vi "Test_Code.vi"() -> ()   [LabVIEW 2015]
uses:
  <instrlib>/Agilent N6700 Series/Agilent N6700 Series.lvlib
  <vilib>/Utility/NIReport.llb/NI_report.lvclass
  Global 5.vi
  <vilib>/Instr/_visa.llb/Select Event Type.ctl
  <vilib>/Instr/_visa.llb/VISA Configure Serial Port (Instr).vi
  Serial - XON-XOFF Characters.ctl
  Serial - ASCII Characters.ctl
  Serial - Settings.ctl
panel:
  in  "report file path":path=path "C:/Users/Tulio/Documents/Testes/Backup excel/backup excel.xlsx"
  out "Hour":i32
  out "Minute":i32
  out "Second":i32
  out "Fractional Second":dbl format="%#.4g"
  in  "Negative Voltage Limit (0.0 volts)":dbl format="%^.3e"
  out "Waveform Graph":dbl[](graph)
  out "Count":i32
  out "read buffer":string
  in  "Read Count":u32=1000
  out "Action":string
  in  "Termination Character":u8=10 format="%.0x"
  in  "End Write on Termination Character?":bool=TRUE
  in  "VISA resource name 2":refnum<visa-resource-name>="COM27"
  in  "XON/XOFF Characters":T1={"XON"=enum."DC1", "XOFF"=enum."DC3"}
  in  "Serial Settings":T3={"baud rate"=9600, "data bits"=8, "parity"=enum."None", "stop bits"=10, "flow control"=0} {"flow control" items=["None"=0, "XON/XOFF"=1, "RTS/CTS"=2, "DTR/DSR"=4]; "stop bits" items=["1.0"=10, "1.5"=15, "2.0"=20]; "data bits" min=5 max=8 step=1; "baud rate" items=["75"=75, "110"=110, "134"=134, "150"=150, "300"=300, "600"=600, "1200"=1200, "1800"=1800, "2400"=2400, "4800"=4800, "7200"=7200, "9600"=9600, "14400"=14400, "19200"=19200, "28800"=28800, "38400"=38400, "56000"=56000, "57600"=57600, "115200"=115200, "128000"=128000, "230400"=230400]}
  in  "End Read on Termination Character?":bool=TRUE
  in  "Start":bool
  in  "Priority (1: Voltage)":i32(ring) items=["Voltage"=1, "Current"=0]
  out "Current Measurement":dbl format="%^.3e"
  in  "Positive Voltage Limit  (5.0 V)":dbl=5.0 format="%^.3e"
  in  "Channel Name (1)":string="4"
  in  "VISA resource name":refnum<visa-resource-name>="USB0::0x0957::0x0F07::MY53002228::INSTR"
  in  "stop":bool
  # "SERIAL"
  # "POWER ANALYZER"
  # "EXCEL"
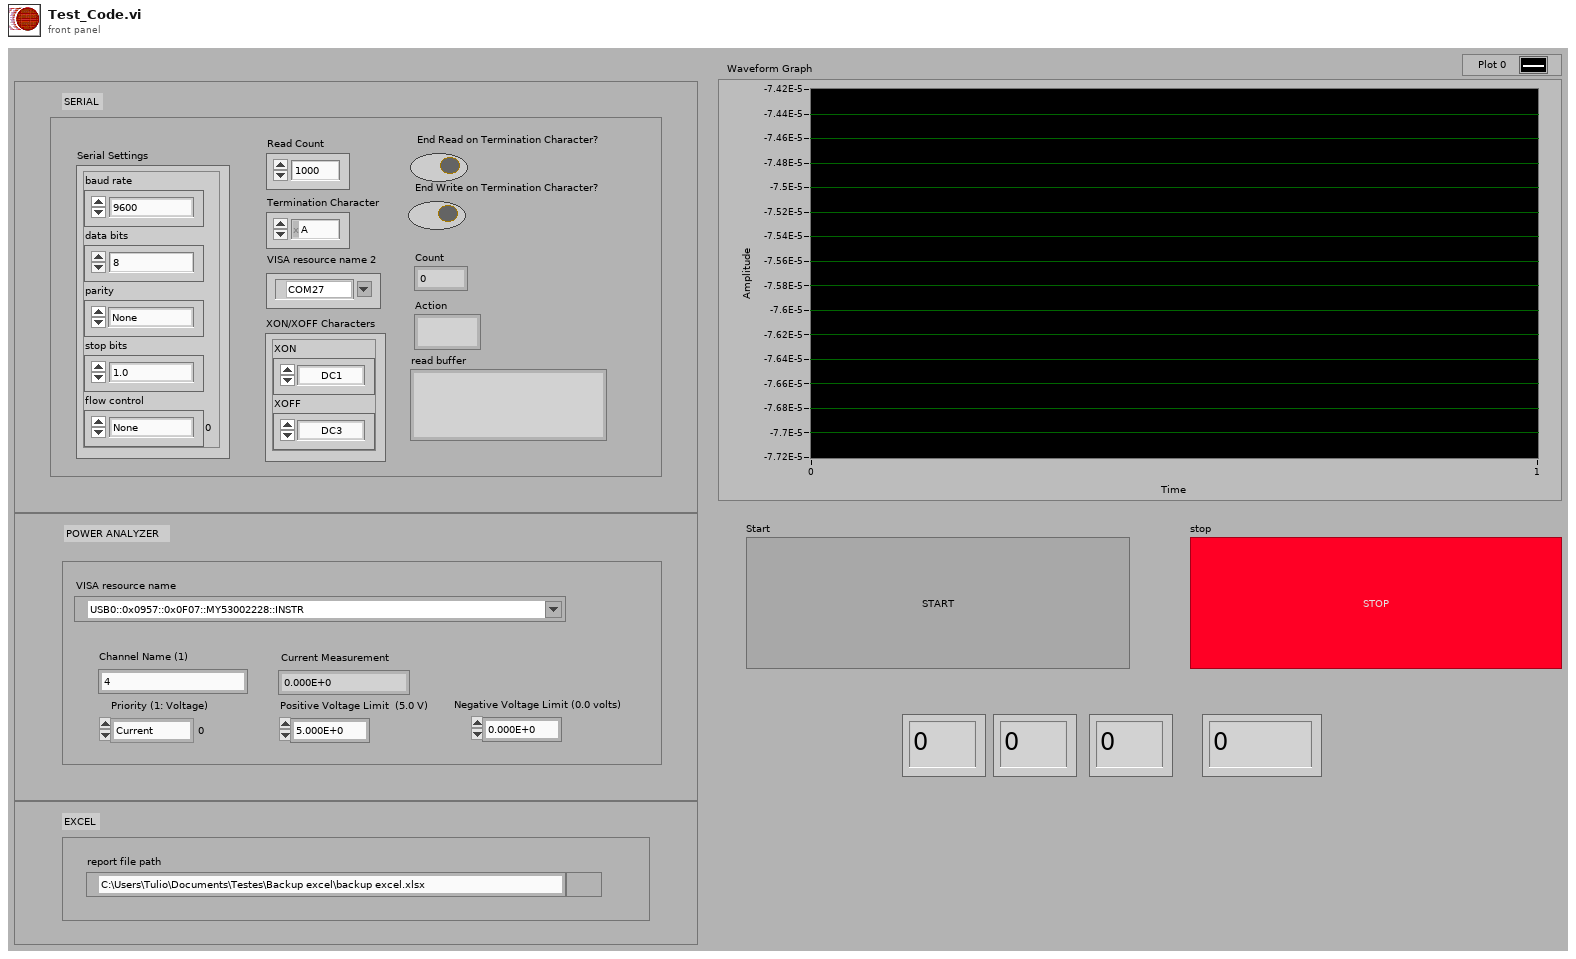
[diagram p1: front panel]
types:
  T1 = typedef "Serial - XON-XOFF Characters.ctl" = cluster{"XON":T2, "XOFF":T2}
  T2 = typedef "Serial - ASCII Characters.ctl" = enum16{"NUL", "SOH", "STX", "ETX", "EOT", "ENQ", "ACK", "BEL", "BS", "HT", "LF", "VT", "FF", "CR", "SO", "SI", "DLE", "DC1", "DC2", "DC3", "DC4", "NAK", "SYN", "ETB", "CAN", "EM", "SUB", "ESC", "FS", "GS", "RS", "US", "SP", "!", "\"", "#", "$", "%", "&", "'", "(", ")", "*", "+", ",", "- (-)", ".", "/", "0", "1", "2", "3", "4", "5", "6", "7", "8", "9", ":", ";", "<", "=", ">", "?", "@", "A", "B", "C", "D", "E", "F", "G", "H", "I", "J", "K", "L", "M", "N", "O", "P", "Q", "R", "S", "T", "U", "V", "W", "X", "Y", "Z", "[", "\\", "]", "^", "_", "`", "a", "b", "c", "d", "e", "f", "g", "h", "i", "j", "k", "l", "m", "n", "o", "p", "q", "r", "s", "t", "u", "v", "w", "x", "y", "z", "{", "|", "}", "~"}
  T3 = typedef "Serial - Settings.ctl" = cluster{"baud rate":u32, "data bits":u16, "parity":enum16{"None", "Odd", "Even", "Mark", "Space"}, "stop bits":u16, "flow control":u16}
  T4 = enum16{"Standard Report", "HTML", "Word", "Excel"}
  T5 = typedef "Select Event Type.ctl" = u32
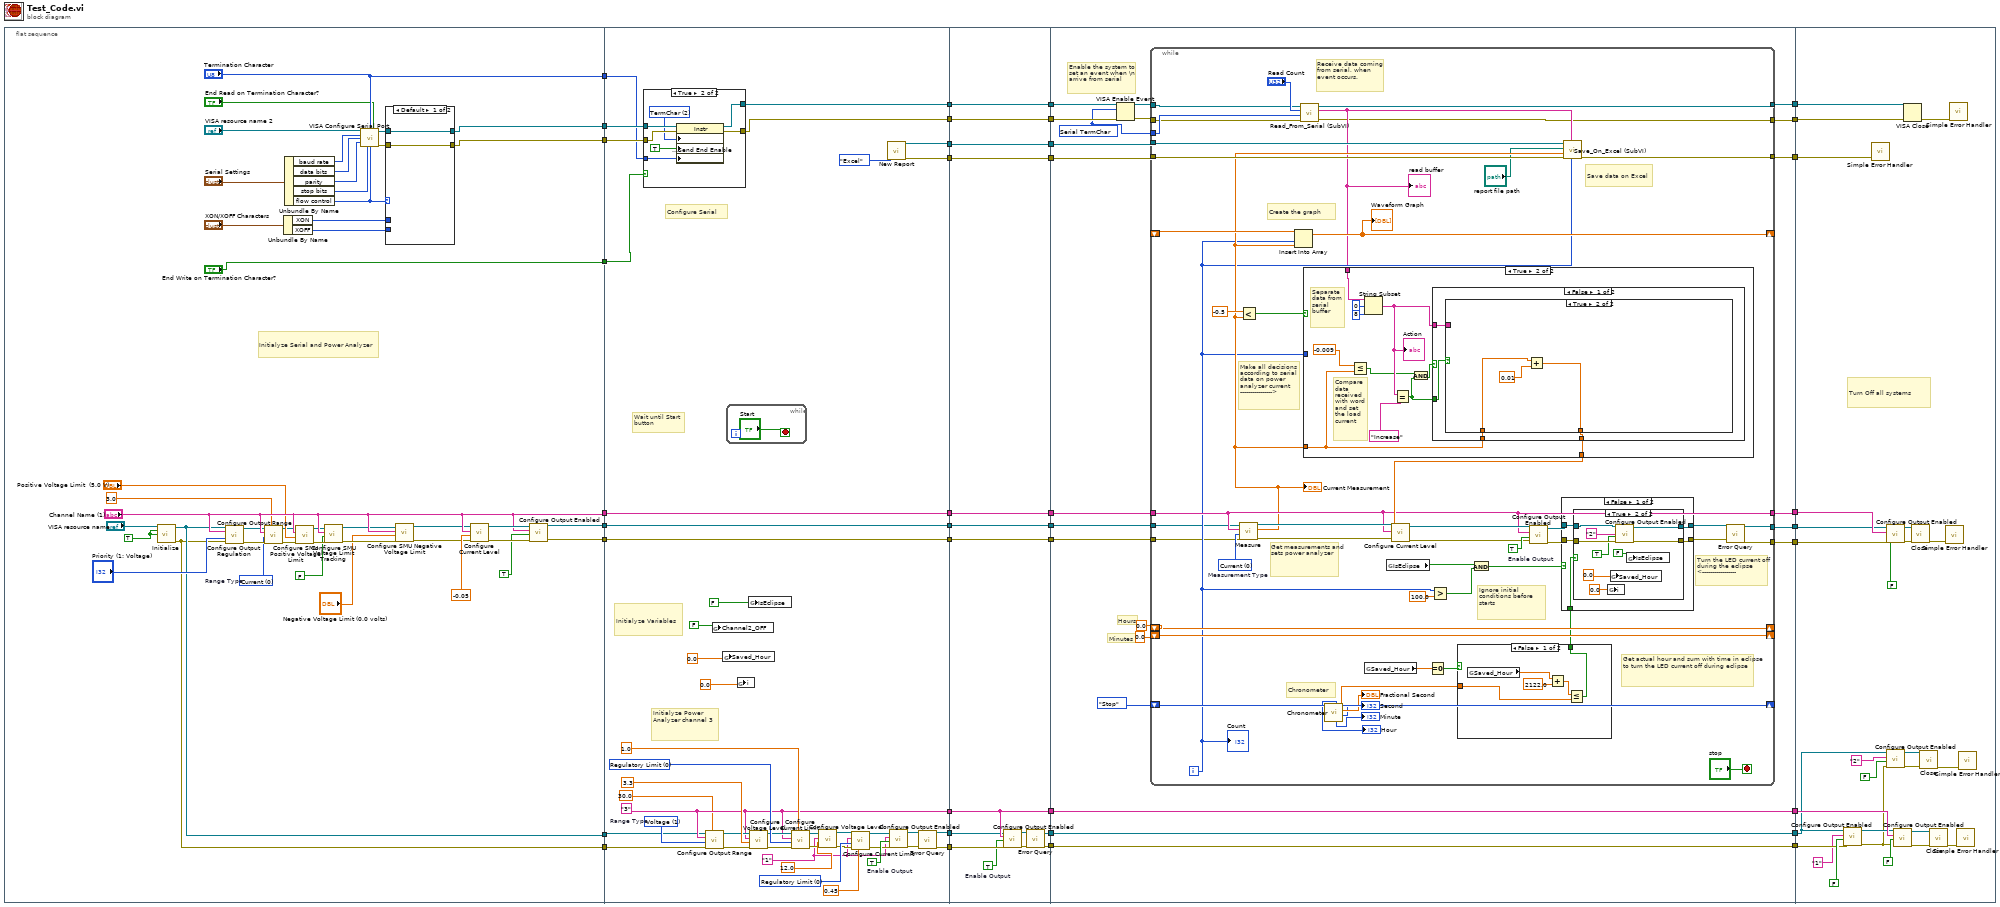
[diagram p0: block diagram]
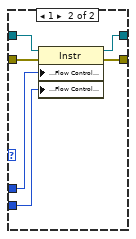
[diagram p2: hidden frame]
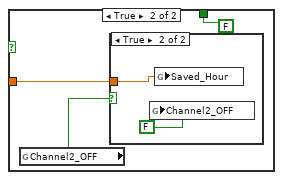
[diagram p4: hidden frame]
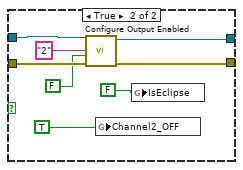
[diagram p7: hidden frame]
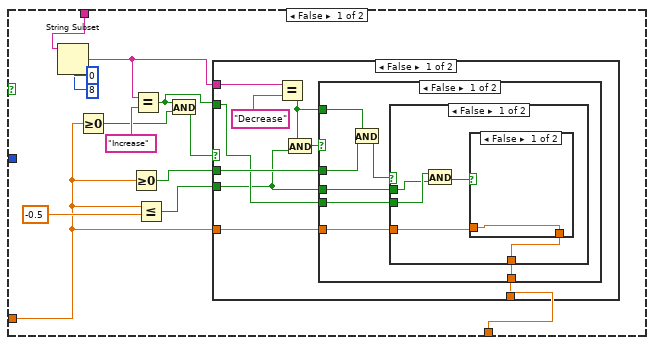
[diagram p8: hidden frame]
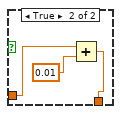
[diagram p9: hidden frame]
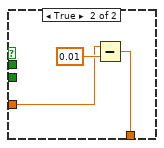
[diagram p10: hidden frame]
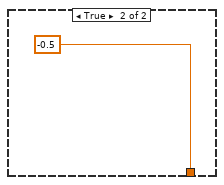
[diagram p11: hidden frame]
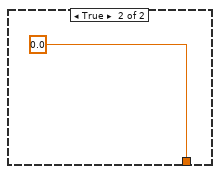
[diagram p12: hidden frame]
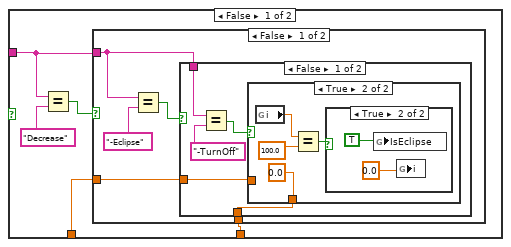
[diagram p13: hidden frame]
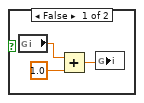
[diagram p15: hidden frame]
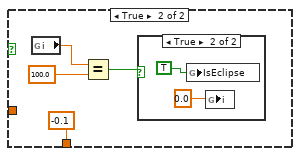
[diagram p16: hidden frame]
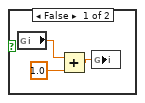
[diagram p17: hidden frame]
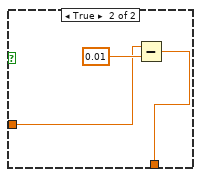
[diagram p18: hidden frame]
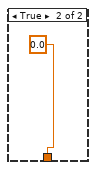
[diagram p19: hidden frame]
diagram:
  n1 = flat-sequence {
    tunnel: ["Channel Name (1)"] -> w38
    tunnel: [w80] -> w37
    tunnel: [w79] -> w36
    tunnel: [w40] -> w35
    tunnel: [w39] -> w34
    tunnel: [w76] -> w25
    tunnel: [w75] -> w24
    tunnel: ["End Write on Termination Character?"] -> w23
    tunnel: ["Termination Character"] -> w22
    tunnel: [w111] -> w20
    tunnel: [w133] -> w18
    tunnel: w38 -> [w133]
    tunnel: [w132] -> w16
    tunnel: w37 -> [w132]
    tunnel: [w131] -> w14
    tunnel: w36 -> [w131]
    tunnel: w35 -> [w112]
    tunnel: w34 -> [w114]
    tunnel: [w122] -> w11
    tunnel: w25 -> [w121]
    tunnel: w24 -> [w120]
    tunnel: w23 -> [w119]
    tunnel: w22 -> [w118]
    tunnel: [w110] -> w9
    tunnel: [w116] -> w7
    tunnel: [w115] -> w5
    tunnel: [w92] -> w2
    tunnel: [w91] -> w1
    tunnel: w20 -> [w158]
    tunnel: [w158] -> w19
    tunnel: w18 -> [w157]
    tunnel: [w157] -> w17
    tunnel: w16 -> [w156]
    tunnel: [w156] -> w15
    tunnel: w14 -> [w155]
    tunnel: [w155] -> w13
    tunnel: [w150] -> w12
    tunnel: w11 -> [w145]
    tunnel: [w145] -> w10
    tunnel: w9 -> [w154]
    tunnel: [w154] -> w8
    tunnel: w7 -> [w153]
    tunnel: [w153] -> w6
    tunnel: w5 -> [w152]
    tunnel: [w152] -> w4
    tunnel: [w151] -> w3
    tunnel: w2 -> [w144]
    tunnel: w1 -> [w147]
    tunnel: w19 -> [w164]
    tunnel: w17 -> [w180]
    tunnel: w15 -> [w179]
    tunnel: w13 -> [w178]
    tunnel: [w177] -> w33
    tunnel: [w176] -> w32
    tunnel: [w175] -> w31
    tunnel: [w174] -> w30
    tunnel: [w173] -> w29
    tunnel: w12 -> [w173]
    tunnel: w10 -> [w172]
    tunnel: [w172] -> w28
    tunnel: [w159] -> w27
    tunnel: [w171] -> w26
    tunnel: w8 -> [w163]
    tunnel: w6 -> [w167]
    tunnel: w4 -> [w166]
    tunnel: [w165] -> w21
    tunnel: w3 -> [w174]
    tunnel: w26 -> [w378]
    tunnel: w27 -> [w379]
    tunnel: w28 -> [w381]
    tunnel: w29 -> [w366]
    tunnel: w30 -> [w368]
    tunnel: w31 -> [w386]
    tunnel: w32 -> [w371]
    tunnel: w33 -> [w370]
    tunnel: w21 -> [w372]
    frame #0 {
      w65 = TRUE ("Reset? (T: Yes)")
      w64 = 0 items=["Voltage"=1, "Current"=0]  # Range Type
      # "Initialyze Serial and Power Analyzer"
      n2 = call <instrlib>:"Initialize.vi"("VISA resource name"="VISA resource name", "ID Query? (T: Yes)"=w65, "Reset? (T: Yes)"=w65) -> ("VISA resource name out"=w40:refnum<visa-resource-name>, "error out"=w39:errorcluster)  [unwired: 11 in]
      n3 = call <instrlib>:"Configure Output Regulation.vi"("VISA resource name"=w40, "Channel Name (1)"="Channel Name (1)", "Output Regulation Priority (1: Voltage)"="Priority (1: Voltage)", "error in (no error)"=w39) -> ("VISA resource name out"=w66:refnum<visa-resource-name>, "error out"=w67:errorcluster)  [unwired: 10 in]
      n4 = call <instrlib>:"Configure Output Range.vi"("Range (0.0)"=3.0, "error in (no error)"=w67, "Range Type (1: Voltage)"=w64, "Channel Name (1)"="Channel Name (1)", "VISA resource name"=w66) -> ("error out"=w69:errorcluster, "VISA resource name out"=w68:refnum<visa-resource-name>)  [unwired: 5 in]
      n5 = Unbundle By Name("XON/XOFF Characters") -> ("XON"=w57:T2, "XOFF"=w58:T2)
      n6 = Unbundle By Name("Serial Settings") -> ("baud rate"=w53:u32, "data bits"=w52:u16, "parity"=w51:enum16{"None", "Odd", "Even", "Mark", "Space"}, "stop bits"=w50:u16, "flow control"=w56:u16)
      n7 = call <instrlib>:"Configure SMU Positive Voltage Limit.vi"("error in (no error)"=w69, "Positive Voltage Limit (0.0 volts)"="Positive Voltage Limit  (5.0 V)", "Channel Name (1)"="Channel Name (1)", "VISA resource name"=w68) -> ("error out"=w71:errorcluster, "VISA resource name out"=w70:refnum<visa-resource-name>)  [unwired: 6 in]
      n8 = call <instrlib>:"Configure SMU Voltage Limit Tracking.vi"("error in (no error)"=w71, "Enable Voltage Limit Tracking (False)"=FALSE, "Channel Name (1)"="Channel Name (1)", "VISA resource name"=w70) -> ("error out"=w44:errorcluster, "VISA resource name out"=w45:refnum<visa-resource-name>)  [unwired: 6 in]
      n9 = call-poly "VISA Configure Serial Port"("VISA resource name"="VISA resource name 2", "termination char\n(0xA = '\\n' = LF)"="Termination Character", "Enable Termination\nChar (T)"="End Read on Termination Character?", "baud rate (9600)"=w53, "data bits (8)"=w52, "parity (0:none)"=w51, "stop bits (10: 1 bit)"=w50, "flow control (0:none)"=w56) -> ("VISA resource name out"=w49:refnum<visa-resource-name>, "error out"=w48:errorcluster)  [unwired: 2 in, 4 out]
      n10 = case shown="Default" w56 {
        tunnel: [w83 w90] -> w75
        tunnel: [w84 w89] -> w76
        tunnel: w48 -> [w83 w88]
        tunnel: w49 -> [w84 w87]
        tunnel: w57 -> [_ w86]
        tunnel: w58 -> [_ w85]
        frame Default {
        }
        frame 1 {
          n11 = property class="Instr"(reference=w87, error in=w88, "Serial Settings:Flow Control XON Character"=w86, "Serial Settings:Flow Control XOFF Character"=w85) -> (reference out=w89:refnum<visa-resource-name>, error out=w90:errorcluster)
        }
      }
      n12 = call <instrlib>:"Configure SMU Negative Voltage Limit.vi"("error in (no error)"=w44, "Negative Voltage Limit (0.0 volts)"="Negative Voltage Limit (0.0 volts)", "Channel Name (1)"="Channel Name (1)", "VISA resource name"=w45) -> ("error out"=w41:errorcluster, "VISA resource name out"=w42:refnum<visa-resource-name>)  [unwired: 6 in]
      n13 = call <instrlib>:"Configure Current Level.vi"("error in (no error)"=w41, "Level  (0.0 A)"=-0.05, "Channel Name (1)"="Channel Name (1)", "VISA resource name"=w42) -> ("error out"=w81:errorcluster, "VISA resource name out"=w82:refnum<visa-resource-name>)  [unwired: 6 in]
      n14 = call <instrlib>:"Configure Output Enabled.vi"("error in (no error)"=w81, "Enable Output (False)"=TRUE, "Channel Name (1)"="Channel Name (1)", "VISA resource name"=w82) -> ("error out"=w79:errorcluster, "VISA resource name out"=w80:refnum<visa-resource-name>)  [unwired: 6 in]
    }
    frame #1 {
      w94 = "1" ("Channel Name (1)")
      w102 = 0 items=["Regulatory Limit", "Trip Limit"] ("Behavior (0: Regulatory Limit)")
      w104 = TRUE  # Enable Output
      w122 = "3" ("Channel Name (1)")
      w129 = 0 items=["Regulatory Limit", "Trip Limit"] ("Behavior (0: Regulatory Limit)")
      w125 = 1 items=["Voltage"=1, "Current"=0]  # Range Type
      # "Initialyze Power Analyzer channel 3"
      # "Initialyze Variables"
      # "Wait until Start button"
      # "Configure Serial"
      n15 = case shown="True" w119 {
        tunnel: w121 -> [w134 w142]
        tunnel: w120 -> [w135 w141]
        tunnel: [w134 w140] -> w111
        tunnel: [w135 w139] -> w110
        tunnel: w118 -> [_ w137]
        frame False {
        }
        frame True {
          w138 = u16 2 items=["None", "LastBit", "TermChar", "Break"] ("Serial Settings:Serial End Mode for Writes")
          n16 = property class="Instr"(reference=w142, error in=w141, "Serial Settings:End Mode for Writes"=w138, "Message Based Settings:Send End Enable"=TRUE, "Message Based Settings:Termination Character"=w137) -> (reference out=w140:refnum<visa-resource-name>, error out=w139:errorcluster)
        }
      }
      n17 = call <instrlib>:"Configure Output Range.vi"("Range (0.0)"=30.0, "error in (no error)"=w114, "Range Type (1: Voltage)"=w125, "Channel Name (1)"=w122, "VISA resource name"=w112) -> ("error out"=w127:errorcluster, "VISA resource name out"=w126:refnum<visa-resource-name>)  [unwired: 5 in]
      n18 = global write "Global 5.vi" "Channel2_OFF"(FALSE ("Boolean")) -> ()
      n19 = global write "Global 5.vi" "Saved_Hour"(0.0 ("Numeric")) -> ()
      n20 = while {
        stop <- "Start" stop-if-true
      }
      n21 = global write "Global 5.vi" "i"(0.0 ("i")) -> ()
      n22 = global write "Global 5.vi" "IsEclipse"(FALSE ("Boolean")) -> ()
      n23 = call <instrlib>:"Configure Voltage Level.vi"("error in (no error)"=w127, "Level  (0.0 volts)"=3.3, "Channel Name (1)"=w122, "VISA resource name"=w126) -> ("error out"=w123:errorcluster, "VISA resource name out"=w124:refnum<visa-resource-name>)  [unwired: 6 in]
      n24 = call <instrlib>:"Configure Current Limit.vi"("Limit (0.0 amps)"=1.0, "error in (no error)"=w123, "Behavior (0: Regulatory Limit)"=w129, "Channel Name (1)"=w122, "VISA resource name"=w124) -> ("error out"=w98:errorcluster, "VISA resource name out"=w97:refnum<visa-resource-name>)  [unwired: 5 in]
      n25 = call <instrlib>:"Configure Voltage Level.vi"("error in (no error)"=w98, "Level  (0.0 volts)"=12.0, "Channel Name (1)"=w94, "VISA resource name"=w97) -> ("error out"=w99:errorcluster, "VISA resource name out"=w100:refnum<visa-resource-name>)  [unwired: 6 in]
      n26 = call <instrlib>:"Configure Current Limit.vi"("Limit (0.0 amps)"=0.45, "error in (no error)"=w99, "Behavior (0: Regulatory Limit)"=w102, "Channel Name (1)"=w94, "VISA resource name"=w100) -> ("error out"=w95:errorcluster, "VISA resource name out"=w96:refnum<visa-resource-name>)  [unwired: 5 in]
      n27 = call <vilib>:"New Report.vi"("report type"=T4."Excel") -> ("report out"=w116:refnum<class "NI_report.lvclass">, "error out"=w115:errorcluster)  [unwired: 13 in]
      n28 = call <instrlib>:"Configure Output Enabled.vi"("error in (no error)"=w95, "Enable Output (False)"=w104, "Channel Name (1)"=w94, "VISA resource name"=w96) -> ("error out"=w105:errorcluster, "VISA resource name out"=w93:refnum<visa-resource-name>)  [unwired: 6 in]
      n29 = call <instrlib>:"Error Query.vi"("VISA resource name"=w93, "error in (no error)"=w105) -> ("VISA resource name out"=w92:refnum<visa-resource-name>, "error out"=w91:errorcluster)  [unwired: 10 in, 2 out]
    }
    frame #2 {
      w146 = TRUE  # Enable Output
      n30 = call <instrlib>:"Configure Output Enabled.vi"("error in (no error)"=w147, "Enable Output (False)"=w146, "Channel Name (1)"=w145, "VISA resource name"=w144) -> ("error out"=w149:errorcluster, "VISA resource name out"=w148:refnum<visa-resource-name>)  [unwired: 6 in]
      n31 = call <instrlib>:"Error Query.vi"("VISA resource name"=w148, "error in (no error)"=w149) -> ("VISA resource name out"=w151:refnum<visa-resource-name>, "error out"=w150:errorcluster)  [unwired: 10 in, 2 out]
    }
    frame #3 {
      w160 = T5 1073684516 items=["Service Request"=1073684491, "Trigger"=3221168138, "Clear"=1073684493, "VXI Signal"=1073684512, "VXI/VME Interrupt"=3221168161, "VXI/VME Sysfail"=1073684509, "VXI/VME Sysreset"=1073684510, "GPIB CIC"=1073684498, "GPIB Talk"=1073684499, "GPIB Listen"=1073684500, "PXI Interrupt"=1073684514, "Serial Break"=1073684515, "Serial TermChar"=1073684516, "Serial CTS"=1073684521, "Serial DSR"=1073684522, "Serial DCD"=1073684524, "Serial RI"=1073684526, "Serial Character"=1073684533, "USB Interrupt"=1073684535, "All Enabled"=1073709055] ("Event Type")
      # "Enable the system to set an event when \\n arrive from serial"
      # "Minutes"
      # "Hours"
      n32 = VISA Enable Event(8:w163, 10:w160, 11:w164) -> (0:w162:errorcluster, 3:w161:refnum<visa-resource-name>)  [unwired: 1 in]
      n33 = while {
        tunnel: w161 -> [w191]
        tunnel: w180 -> [w221]
        tunnel: w179 -> [w193]
        tunnel: w178 -> [w192]
        tunnel: [w206] -> w177
        tunnel: [w207] -> w176
        tunnel: [w221] -> w175
        tunnel: [w189] -> w171
        tunnel: w162 -> [w187]
        shift-right: [w217] -> _
        shift-left: enum16{"Count", "Stop", "Reset"}."Stop" ("Action") -> [w218]
        shift-right: [w216] -> _
        shift-left: 0.0 -> [w216]
        shift-right: [w215] -> _
        shift-left: 0.0 -> [w215]
        tunnel: w167 -> [w214]
        tunnel: w166 -> [w213]
        tunnel: [w209] -> w165
        shift-right: [w212] -> _
        shift-left: _ -> [w211]
        tunnel: w160 -> [w190]
        tunnel: [w188] -> w159
        i -> [w201]
        stop <- "stop" stop-if-true
        w225 = 0 items=["Voltage"=1, "Current"=0]  # Measurement Type
        w228 = TRUE  # Enable Output
        # "Ignore initial conditions before starts"
        # "Turn the LED current off during the eclipse \n<-----------------"
        # "Get actual hour and sum with time in eclipse to turn the LED current off during eclipse"
        # "Chronometer"
        # "Get measurements and sets power analyzer"
        # "Make all decisions according to serial data on power analyzer current\n---------------->"
        # "Create the graph"
        # "Save data on Excel"
        # "Receive data coming from serial, when event occurs."
        n34 = call <instrlib>:"Measure.vi"("error in (no error)"=w192, "Measurement Type (1: Voltage)"=w225, "Channel Name (1)"=w221, "VISA resource name"=w193) -> ("error out"=w222:errorcluster, "Measurement"=w210:dbl, "VISA resource name out"=w223:refnum<visa-resource-name>)  [unwired: 5 in]
        "Current Measurement" <- w210
        n35 = Less?(x=-0.5, y=w210) -> (x < y?=w220:bool)
        n36 = Insert Into Array(array=w211, index=w201, new element=w210) -> (w212:dbl[])
        "Waveform Graph" <- w212
        n37 = call "Read_From_Serial (SubVI).vi"("error in (no error)"=w187, "Event Type"=w190, "Read Count"="Read Count", "VISA Refnum in"=w191) -> ("error out"=w189:errorcluster, "read buffer"=w194:string, "VISA Refnum out"=w188:refnum<visa-resource-name>)  [unwired: 5 in]
        "read buffer" <- w194
        n38 = case shown="True" w220 {
          tunnel: [w277 w318] -> w224
          tunnel: w210 -> [w266 w311]
          tunnel: w194 -> [w270 w316]
          tunnel: w201 -> [_ _]
          frame False {
            n39 = String Subset(string=w270, offset (0)=0, length (rest)=8 ("length (rest)")) -> (substring=w269:string)
            n40 = Greater Or Equal To 0?(x=w266) -> (x >= 0?=w265:bool)
            n41 = Greater Or Equal To 0?(x=w266) -> (x >= 0?=w268:bool)
            n42 = Equal?(x=w269, y="Increase") -> (x = y?=w267:bool)
            n43 = Less Or Equal?(x=w266, y=-0.5) -> (x <= y?=w274:bool)
            n44 = And(x=w267, y=w265) -> (x .and. y?=w276:bool)
            n45 = case shown="False" w276 {
              tunnel: [w283 0.0] -> w277
              tunnel: w274 -> [w278 _]
              tunnel: w269 -> [w285 _]
              tunnel: w268 -> [w281 _]
              tunnel: w266 -> [w280 _]
              tunnel: w267 -> [w279 _]
              frame False {
                n46 = Equal?(x=w285, y="Decrease") -> (x = y?=w282:bool)
                n47 = And(x=w282, y=w278) -> (x .and. y?=w286:bool)
                n48 = case shown="False" w286 {
                  tunnel: [w290 -0.5] -> w283
                  tunnel: w282 -> [w292 _]
                  tunnel: w281 -> [w291 _]
                  tunnel: w280 -> [w289 _]
                  tunnel: w279 -> [w288 _]
                  tunnel: w278 -> [w287 _]
                  frame False {
                    n49 = And(x=w292, y=w291) -> (x .and. y?=w293:bool)
                    n50 = case shown="False" w293 {
                      tunnel: [w295 w305] -> w290
                      tunnel: w289 -> [w294 w303]
                      tunnel: w288 -> [w298 _]
                      tunnel: w287 -> [w297 _]
                      frame False {
                        n51 = And(x=w298, y=w297) -> (x .and. y?=w296:bool)
                        n52 = case shown="False" w296 {
                          tunnel: [w299 w302] -> w295
                          tunnel: w294 -> [w299 w301]
                          frame False {
                          }
                          frame True {
                            n53 = Add(x=w301, y=0.01) -> (x+y=w302:dbl)
                          }
                        }
                      }
                      frame True {
                        n54 = Subtract(x=w303, y=0.01) -> (x-y=w305:dbl)
                      }
                    }
                  }
                  frame True {
                  }
                }
              }
              frame True {
              }
            }
          }
          frame True {
            # "Compare data received with word and set the load current"
            # "Separate data from serial buffer"
            n55 = Less Or Equal?(x=-0.009, y=w311) -> (x <= y?=w308:bool)
            n56 = String Subset(string=w316, offset (0)=0, length (rest)=8 ("length (rest)")) -> (substring=w313:string)
            "Action" <- w313
            n57 = Equal?(x=w313, y="Increase") -> (x = y?=w310:bool)
            n58 = And(x=w308, y=w310) -> (x .and. y?=w309:bool)
            n59 = case shown="False" w309 {
              tunnel: [w322 0.0 ("Measurement")] -> w318
              tunnel: w310 -> [w321 _]
              tunnel: w311 -> [w320 _]
              tunnel: w313 -> [w319 _]
              frame False {
                n60 = case shown="True" w321 {
                  tunnel: [w327 w361] -> w322
                  tunnel: w319 -> [w323 _]
                  tunnel: w320 -> [w324 w360]
                  frame False {
                    n61 = Equal?(x=w323, y="Decrease") -> (x = y?=w326:bool)
                    n62 = case shown="False" w326 {
                      tunnel: [w330 w358] -> w327
                      tunnel: w324 -> [w329 w357]
                      tunnel: w323 -> [w328 _]
                      frame False {
                        n63 = Equal?(x=w328, y="-Eclipse") -> (x = y?=w332:bool)
                        n64 = case shown="False" w332 {
                          tunnel: [w334 -0.1] -> w330
                          tunnel: w329 -> [w333 _]
                          tunnel: w328 -> [w336 _]
                          frame False {
                            n65 = Equal?(x=w336, y="-TurnOff") -> (x = y?=w337:bool)
                            n66 = case shown="True" w337 {
                              tunnel: [w338 0.0 ("x")] -> w334
                              tunnel: w333 -> [w338 _]
                              frame False {
                              }
                              frame True {
                                n67 = global read "Global 5.vi" "i"() -> (w339:dbl)
                                n68 = Equal?(x=w339, y=100.0) -> (x = y?=w341:bool)
                                n69 = case shown="True" w341 {
                                frame False {
                                n70 = global read "Global 5.vi" "i"() -> (w343:dbl)
                                n71 = Add(x=w343, y=1.0) -> (x+y=w344:dbl)
                                n72 = global write "Global 5.vi" "i"(w344) -> ()
                                }
                                frame True {
                                n73 = global write "Global 5.vi" "IsEclipse"(TRUE ("Boolean")) -> ()
                                n74 = global write "Global 5.vi" "i"(0.0 ("i")) -> ()
                                }
                                }
                              }
                            }
                          }
                          frame True {
                            n75 = global read "Global 5.vi" "i"() -> (w348:dbl)
                            n76 = Equal?(x=w348, y=100.0) -> (x = y?=w350:bool)
                            n77 = case shown="True" w350 {
                              frame False {
                                n78 = global read "Global 5.vi" "i"() -> (w353:dbl)
                                n79 = Add(x=w353, y=1.0) -> (x+y=w352:dbl)
                                n80 = global write "Global 5.vi" "i"(w352) -> ()
                              }
                              frame True {
                                n81 = global write "Global 5.vi" "IsEclipse"(TRUE ("Boolean")) -> ()
                                n82 = global write "Global 5.vi" "i"(0.0 ("i")) -> ()
                              }
                            }
                          }
                        }
                      }
                      frame True {
                        n83 = Subtract(x=w357, y=0.01) -> (x-y=w358:dbl)
                      }
                    }
                  }
                  frame True {
                    n84 = Add(x=w360, y=0.01) -> (x+y=w361:dbl)
                  }
                }
              }
              frame True {
              }
            }
          }
        }
        n85 = call "Chronometer.vi"("Action in"=w218) -> ("Second"=→"Second":i32, "Fractional Second"=→"Fractional Second":dbl, "Time"=w199:dbl, "Minute"=→"Minute":i32, "Hour"=→"Hour":i32, "Action out"=w217:enum16{"Count", "Stop", "Reset"})  [unwired: 5 in]
        n86 = global read "Global 5.vi" "Saved_Hour"() -> (w185:dbl)
        n87 = global read "Global 5.vi" "IsEclipse"() -> (w186:bool)
        n88 = call <instrlib>:"Configure Current Level.vi"("error in (no error)"=w222, "Level  (0.0 A)"=w224, "Channel Name (1)"=w221, "VISA resource name"=w223) -> ("error out"=w226:errorcluster, "VISA resource name out"=w227:refnum<visa-resource-name>)  [unwired: 6 in]
        n89 = Equal To 0?(x=w185) -> (x = 0?=w198:bool)
        n90 = Greater?(x=w201, y=100.0) -> (0:w203:bool)
        n91 = case shown="False" w198 {
          tunnel: w199 -> [w232 w237]
          tunnel: [w234 FALSE] -> w195
          frame False {
            n92 = global read "Global 5.vi" "Saved_Hour"() -> (w231:dbl)
            n93 = Add(x=w231, y=2122.0) -> (x+y=w233:dbl)
            n94 = Less Or Equal?(x=w233, y=w232) -> (x <= y?=w234:bool)
          }
          frame True {
            n95 = global read "Global 5.vi" "Channel2_OFF"() -> (w238:bool)
            n96 = case shown="True" w238 {
              tunnel: w237 -> [_ w239]
              frame False {
              }
              frame True {
                n97 = global write "Global 5.vi" "Channel2_OFF"(FALSE ("Channel2")) -> ()
                n98 = global write "Global 5.vi" "Saved_Hour"(w239) -> ()
              }
            }
          }
        }
        n99 = And(x=w186, y=w203) -> (x .and. y?=w200:bool)
        n100 = call <instrlib>:"Configure Output Enabled.vi"("error in (no error)"=w226, "Enable Output (False)"=w228, "Channel Name (1)"=w221, "VISA resource name"=w227) -> ("error out"=w204:errorcluster, "VISA resource name out"=w205:refnum<visa-resource-name>)  [unwired: 6 in]
        n101 = case shown="False" w200 {
          tunnel: w205 -> [w244 w263]
          tunnel: w204 -> [w245 w262]
          tunnel: [w242 w260] -> w196
          tunnel: [w243 w259] -> w197
          tunnel: w195 -> [w241 _]
          frame False {
            n102 = case shown="True" w241 {
              tunnel: w244 -> [w246 w251]
              tunnel: w245 -> [w247 w255]
              tunnel: [w247 w253] -> w242
              tunnel: [w246 w252] -> w243
              frame False {
              }
              frame True {
                n103 = global write "Global 5.vi" "i"(0.0 ("i")) -> ()
                n104 = global write "Global 5.vi" "Saved_Hour"(0.0 ("Numeric")) -> ()
                n105 = call <instrlib>:"Configure Output Enabled.vi"("error in (no error)"=w255, "Enable Output (False)"=TRUE, "Channel Name (1)"="2", "VISA resource name"=w251) -> ("error out"=w253:errorcluster, "VISA resource name out"=w252:refnum<visa-resource-name>)  [unwired: 6 in]
                n106 = global write "Global 5.vi" "IsEclipse"(FALSE ("Boolean")) -> ()
              }
            }
          }
          frame True {
            n107 = call <instrlib>:"Configure Output Enabled.vi"("error in (no error)"=w262, "Enable Output (False)"=FALSE, "Channel Name (1)"="2", "VISA resource name"=w263) -> ("error out"=w260:errorcluster, "VISA resource name out"=w259:refnum<visa-resource-name>)  [unwired: 6 in]
            n108 = global write "Global 5.vi" "Channel2_OFF"(TRUE ("Channel2")) -> ()
            n109 = global write "Global 5.vi" "IsEclipse"(FALSE ("Boolean")) -> ()
          }
        }
        n110 = call "Save_On_Excel (SubVI).vi"("Numeric"=w201, "read buffer"=w194, "error in (no error)"=w213, "Measurement"=w210, "report file path"="report file path", "NI_report in"=w214) -> ("error out"=w209:errorcluster)  [unwired: 5 in]
        n111 = call <instrlib>:"Error Query.vi"("VISA resource name"=w197, "error in (no error)"=w196) -> ("VISA resource name out"=w207:refnum<visa-resource-name>, "error out"=w206:errorcluster)  [unwired: 10 in, 2 out]
        "Count" <- w201
      }
    }
    frame #4 {
      # "Turn Off all systems"
      n112 = call <instrlib>:"Configure Output Enabled.vi"("error in (no error)"=w366, "Enable Output (False)"=FALSE, "Channel Name (1)"="1", "VISA resource name"=w368) -> ("error out"=w365:errorcluster, "VISA resource name out"=w367:refnum<visa-resource-name>)  [unwired: 6 in]
      n113 = call <vilib>:"Simple Error Handler.vi"("error in (no error)"=w372) -> ()  [unwired: 1 in, 8 out]
      n114 = call <instrlib>:"Configure Output Enabled.vi"("error in (no error)"=w365, "Enable Output (False)"=FALSE, "Channel Name (1)"="2", "VISA resource name"=w368) -> ("error out"=w376:errorcluster, "VISA resource name out"=w377:refnum<visa-resource-name>)  [unwired: 6 in]
      n115 = call <instrlib>:"Configure Output Enabled.vi"("error in (no error)"=w370, "Enable Output (False)"=FALSE, "Channel Name (1)"=w386, "VISA resource name"=w371) -> ("error out"=w388:errorcluster, "VISA resource name out"=w389:refnum<visa-resource-name>)  [unwired: 6 in]
      n116 = call <instrlib>:"Configure Output Enabled.vi"("error in (no error)"=w365, "Enable Output (False)"=FALSE, "Channel Name (1)"=w381, "VISA resource name"=w367) -> ("error out"=w384:errorcluster, "VISA resource name out"=w383:refnum<visa-resource-name>)  [unwired: 6 in]
      n117 = VISA Close(VISA resource name=w379, error in (no error)=w378) -> (error out=w380:errorcluster)
      n118 = call <instrlib>:"Close.vi"("VISA resource name"=w389, "error in (no error)"=w388) -> ("error out"=w390:errorcluster)  [unwired: 13 in]
      n119 = call <instrlib>:"Close.vi"("VISA resource name"=w377, "error in (no error)"=w376) -> ("error out"=w375:errorcluster)  [unwired: 13 in]
      n120 = call <instrlib>:"Close.vi"("VISA resource name"=w383, "error in (no error)"=w384) -> ("error out"=w385:errorcluster)  [unwired: 13 in]
      n121 = call <vilib>:"Simple Error Handler.vi"("error in (no error)"=w390) -> ()  [unwired: 4 in, 5 out]
      n122 = call <vilib>:"Simple Error Handler.vi"("error in (no error)"=w380) -> ()  [unwired: 1 in, 8 out]
      n123 = call <vilib>:"Simple Error Handler.vi"("error in (no error)"=w385) -> ()  [unwired: 4 in, 5 out]
      n124 = call <vilib>:"Simple Error Handler.vi"("error in (no error)"=w375) -> ()  [unwired: 4 in, 5 out]
    }
  }
